vi "Set Dev Notice Call Back.vi"(8 "error in (no error)":errorcluster, 9 "rmvcallback":cluster{}, 10 "addcallback":cluster{}, 11 "ppara":u32) -> (0 "error out":errorcluster, 3 "ppara out":u32)   [LabVIEW 2021, in "vmmsolib.lvlib"]
doc: "DLL_API void WINAPI SetDevNoticeCallBack(void* ppara, AddCallBack addcallback, RemoveCallBack rmvcallback);"
uses:
  vmmsolib.lvlib
  vmmso.dll
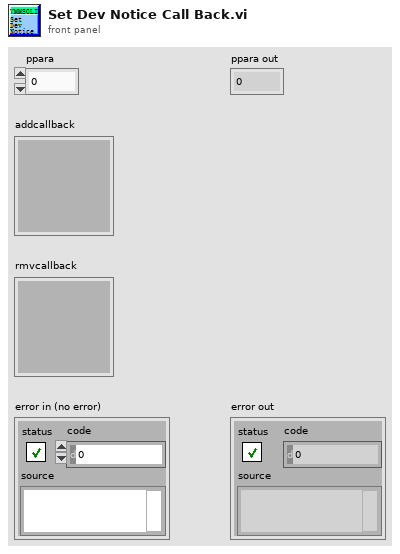
[diagram p1: front panel]
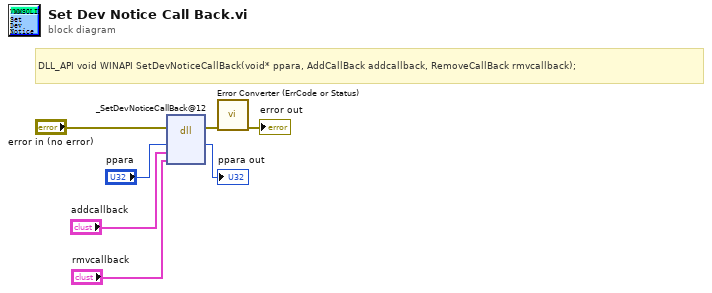
[diagram p0: block diagram]
diagram:
  # "DLL_API void WINAPI SetDevNoticeCallBack(void* ppara, AddCallBack addcallback, RemoveCallBack rmvcallback);"
  n1 = dll-call lib="D:/VmMsoSDK/demo-Labview/2021/vmmsolib/vmmso.*" fn="_SetDevNoticeCallBack@12"(error in="error in (no error)", "ppara"="ppara", "addcallback"="addcallback", "rmvcallback"="rmvcallback") -> (error out=w2:errorcluster, "ppara"=→"ppara out":u32)  [unwired: 5 in, 1 out]
  n2 = call "Error Converter (ErrCode or Status).vi"("error in (no error)"=w2) -> ("error out"=→"error out":errorcluster)  [unwired: 10 in]
